vi "Server Cmd Answer - Get Version.vi"(7 "server event ref":refnum<vi>, 8 "error in":errorcluster, 10 "command header (Get version)":string="Get version") -> (0 "error out":errorcluster, 3 "info data out":string)   [LabVIEW 2020]
doc: "Send answer for command \"Get version\"."
uses:
  octave/infolib/infolib.lvlib
  TWM client/TWM Client.lvlib
  octave/infolib/String.vi
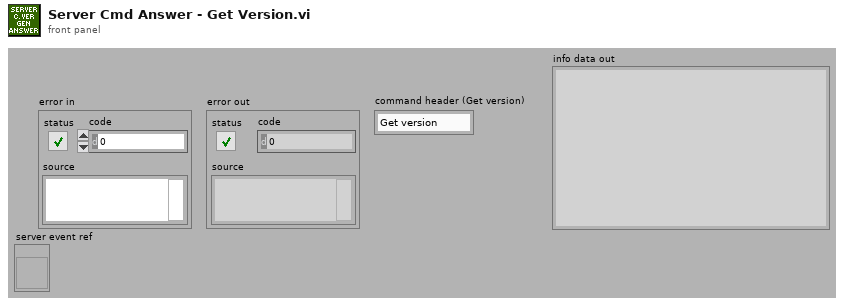
[diagram p1: front panel]
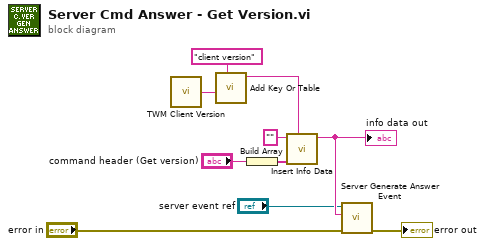
[diagram p0: block diagram]
diagram:
  n1 = call "TWM Client Version.vi"() -> ("version string"=w2:string)
  n2 = call-poly "Add Key Or Table.vi"("key description"="client version", "string"=w2) -> ("info data out"=w1:string)  [unwired: 8 in, 1 out]
  n3 = Build Array("command header (Get version)") -> (w9:string[])
  n4 = call "Insert Info Data.vi"("info data to insert"=w1, "sections"=w9, "info data"="") -> ("info data out"=w7:string)  [unwired: 7 in, 1 out]
  "info data out" <- w7
  n5 = call "Server Generate Answer Event.vi"("error in"="error in", "event data"=w7, "server event ref"="server event ref") -> ("error out"=→"error out":errorcluster)  [unwired: 8 in]
